vi "Conditionning - Truncate wForms.vi"(0 "reference in":refnum<class "GSwFormDSP.lvclass">, 5 "error in (no error)":errorcluster, 6 "Anotate Signal Name":bool=TRUE, 7 "Start (sec)":dbl, 8 "Cut Option":T1(ring), 9 "Duration (sec)":dbl=-1.0) -> (11 "actual start samples/time":dbl format="%_8f", 13 "actual duration":dbl format="%0.2f", 14 "reference in":refnum<class "GSwFormDSP.lvclass">, 19 "error out":errorcluster)   [LabVIEW 2020, in "GSwFormDSP.lvclass"]
uses:
  GSwFormDSP.lvclass
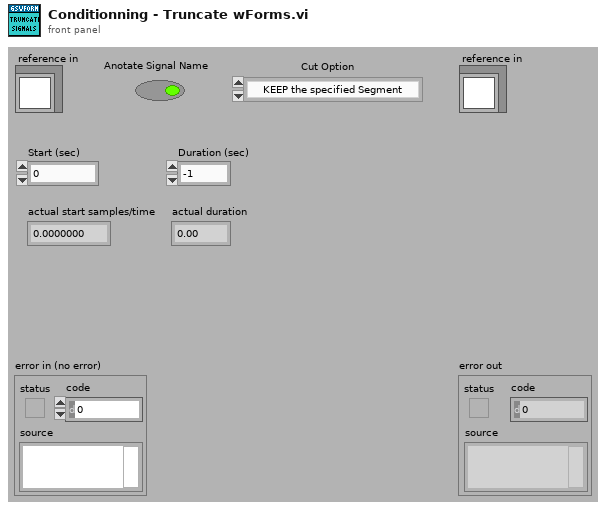
[diagram p1: front panel]
types:
  T1 = enum16{"KEEP the specified Segment", "DELETE the specified Segment"}
  T2 = typedef "GSwFormDSP.lvclass/ObjectAttributesRef.ctl" = refnum<data-value>
  T3 = typedef "GSwFormDSP.lvclass/ObjectAttributes.ctl" = cluster{"Wform Ref":refnum<data-value>, "Nb Signals":i32, "Spectral Function Parameters":T4, "FFT":waveform(cdb)[], "Nb FFT":i32, "Nb Averages":i32[], "Reference Indexes":i32[], "Response Indexes":i32[], "Coherence":waveform(dbl)[], "TDF Parameters":T6, "DAQ":cluster{"Duration (sec)":dbl, "Buffer Size (Samples)":i32, "Offset (Samples)":i32}, "Filter Impulse Response (TDF)":waveform(dbl), "Sound Playback":T7}
  T4 = typedef "GSwFormDSP.lvclass/Spectral Parameters.ctl" = cluster{"Frequency resolution (Hz)":dbl, "Overlap":dbl, "Window":T5}
  T5 = typedef "NI_AALPro.lvlib/windowTd.ctl" = u32
  T6 = typedef "GSwFormDSP.lvclass/TDF Parameters.ctl" = cluster{"Filter":enum32{"Lowpass", "Highpass", "Bandpass", "Bandstop"}, "Type:":enum16{"Butterworth", "Chebyshev", "Inv Chebyshev", "Elliptic", "Bessel"}, "LP cutoff freq":dbl, "HP cutoff freq":dbl, "Order":i32, "passband ripple (dB)":dbl, "stopband attenuation (dB)":dbl, "Phaseless Filter":bool, "Include Fade IN and OUT":bool}
  T7 = typedef "GSwFormDSP.lvclass/Sound Playback.ctl" = cluster{"Timer start (ms)":u32, "task ID":T8, "Cursor Init Location (s)":dbl, "SC Volume":dbl}
  T8 = typedef "Sound Output Task ID.ctl" = u32
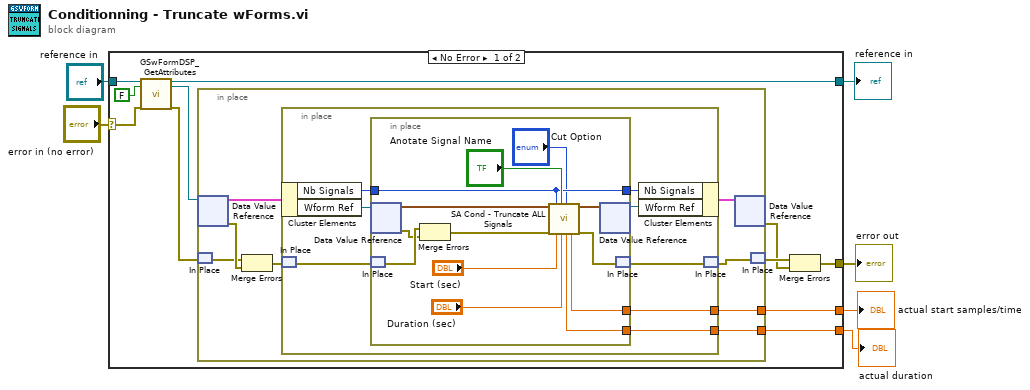
[diagram p0: block diagram]
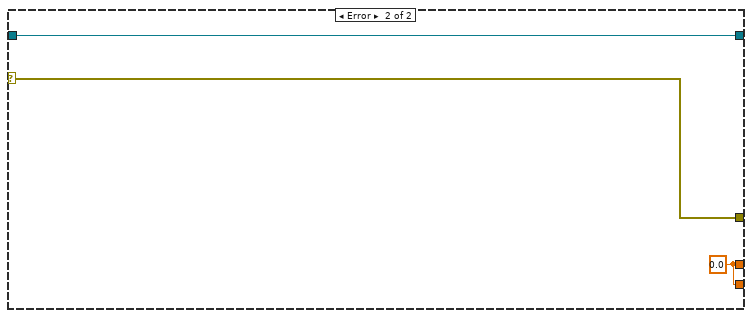
[diagram p2: hidden frame]
diagram:
  n1 = case shown="No Error" "error in (no error)" {
    selector: "error in (no error)" -> [w14 w49]
    tunnel: [w17 w49] -> w5
    tunnel: [w12 w48] -> w3
    tunnel: "reference in" -> [w15 w48]
    tunnel: [w8 w47] -> w2
    tunnel: [w7 w47] -> w1
    frame No Error {
      n2 = call "GSwFormDSP_GetAttributes.vi"("reference in"=w15, "return data? (T)"=FALSE, "error in (no error)"=w14) -> ("reference out"=w12:refnum<class "GSwFormDSP.lvclass">, "attributes ref"=w13:T2, "error out"=w11:errorcluster)  [unwired: 13 in, 1 out]
      n3 = in-place {
        in-place-border: [w19] -> w8
        in-place-border: [w18] -> w7
        n4 = in-place-dvr #1(w13) -> (w23:T3, w25:errorcluster)
        n5 = in-place-match #2(w11) -> (w24:errorcluster)
        n6 = Merge Errors(w24, w25) -> (w22:errorcluster)
        n7 = in-place {
          in-place-border: [w28] -> w19
          in-place-border: [w27] -> w18
          n8 = in-place-cluster #3(w23) -> ("Nb Signals"=w29:i32, "Wform Ref"=w33:refnum<data-value>)
          n9 = in-place-match #4(w22) -> (w31:errorcluster)
          n10 = in-place {
            in-place-border: w29 -> [w35]
            in-place-border: [w37] -> w28
            in-place-border: [w36] -> w27
            in-place-border: [w35] -> w26
            n11 = in-place-dvr #5(w33) -> (w45:waveform(dbl)[], w42:errorcluster)
            n12 = in-place-match #6(w31) -> (w43:errorcluster)
            n13 = Merge Errors(w43, w42) -> (w41:errorcluster)
            n14 = call "SA Cond - Truncate ALL Signals.vi"("wForm IN"=w45, "error in (no error)"=w41, "Nb Signals"=w35, "Start (sec)"="Start (sec)", "Anotate Signal Name"="Anotate Signal Name", "Duration (sec)"="Duration (sec)", "Cut Option"="Cut Option") -> ("actual duration"=w36:dbl, "actual start samples/time"=w37:dbl, "wForm OUT"=w46:waveform(dbl)[], "error out"=w40:errorcluster)  [unwired: 9 in]
            n15 = in-place-dvr #5(w46) -> (w32:refnum<data-value>)  [unwired: 1 out]
            n16 = in-place-match #6(w40) -> (w30:errorcluster)
          }
          n17 = in-place-cluster #3("Nb Signals"=w26, "Wform Ref"=w32) -> (w21:T3)
          n18 = in-place-match #4(w30) -> (w20:errorcluster)
        }
        n19 = in-place-dvr #1(w21) -> (w9:errorcluster)  [unwired: 1 out]
        n20 = in-place-match #2(w20) -> (w10:errorcluster)
      }
      n21 = Merge Errors(w10, w9) -> (w17:errorcluster)
    }
    frame Error {
      w47 = 0.0 ("actual start samples/time")
    }
  }
  "error out" <- w5
  "reference in" <- w3
  "actual start samples/time" <- w2
  "actual duration" <- w1
